vi "QR_code_Check.vi"(5 "Columns":string[](array[string]), 7 "error in (no error)":errorcluster, 8 "replace %s":string, 9 "table":string, 10 "Refnum in":T1) -> (0 "error out":errorcluster, 1 "data":string[][](array[string]), 2 "FALSE healty":bool, 3 "Refnum out":T1, 4 "TRUE Duplication on Station 2":bool)   [LabVIEW 2017]
uses:
  <vilib>/addons/database/Connection.llb/Conn ObjectReference.ctl
  <vilib>/addons/database/NI_Database_API.lvlib
panel:
  out "resulting string":string
  out "PART 1":string
  out "length 2":i32
  out "PART 2":string
  out "length":i32
  out "TRUE no barcode Done on station 1":bool
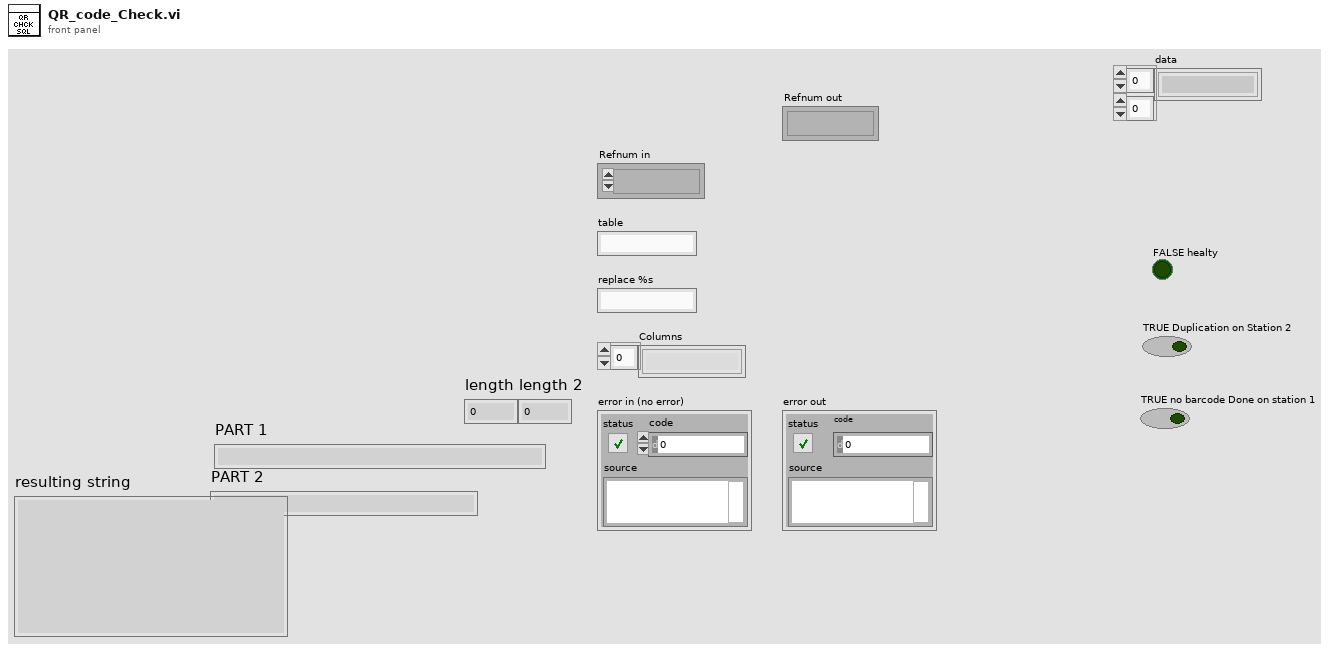
[diagram p1: front panel]
types:
  T1 = typedef "NI_Database_API.lvlib/Conn ObjectReference.ctl" = refnum<k1>
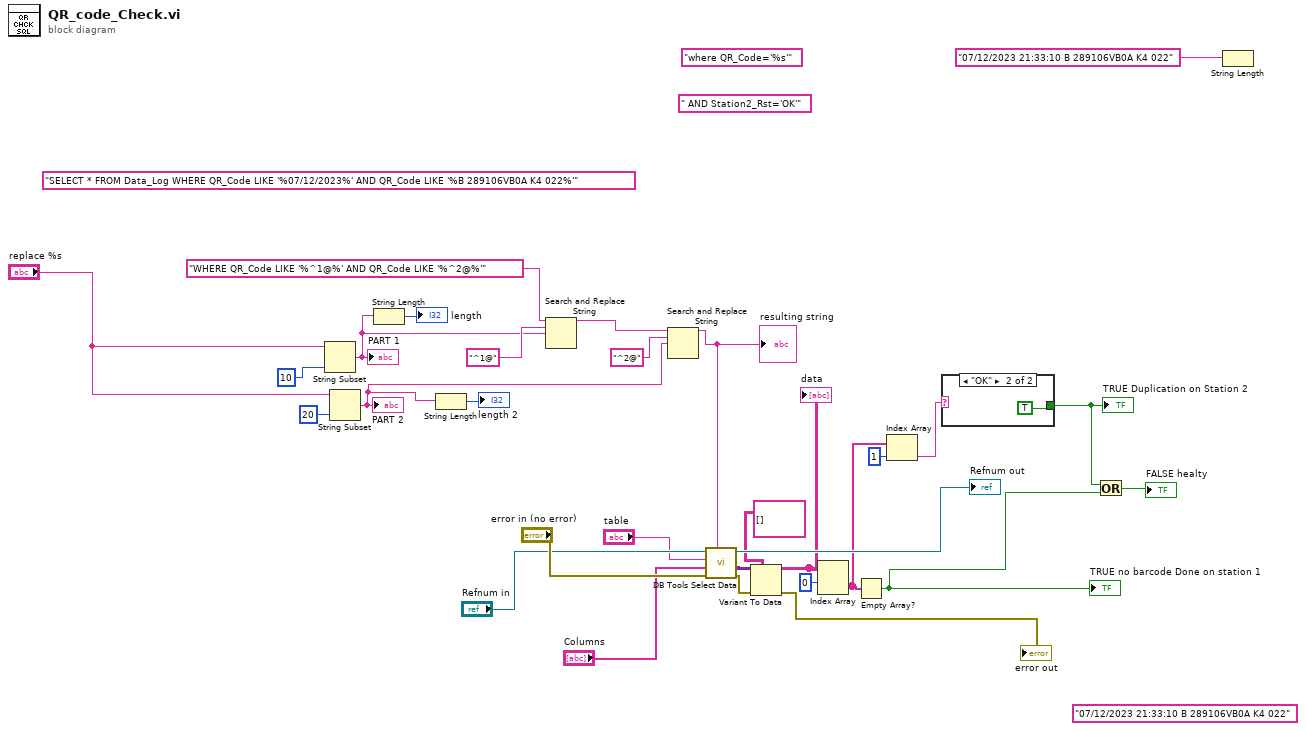
[diagram p0: block diagram]
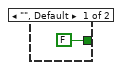
[diagram p2: hidden frame]
diagram:
  (unwired) "07/12/2023 21:33:10 B 289106VB0A K4 022" ("format string")
  (unwired) "SELECT * FROM Data_Log WHERE QR_Code LIKE '%07/12/2023%' AND QR_Code LIKE '%B 289106VB0A K4 022%'" ("format string")
  (unwired) "where QR_Code='%s'" ("format string")
  (unwired) " AND Station2_Rst='OK'" ("replace %s")
  n1 = String Subset(string="replace %s", length (rest)=10 ("offset (0)")) -> (substring=w4:string)  [unwired: 1 in]
  "PART 1" <- w4
  n2 = String Subset(string="replace %s", offset (0)=20) -> (substring=w3:string)  [unwired: 1 in]
  "PART 2" <- w3
  n3 = String Length(string=w4) -> (length=→"length":i32)
  n4 = String Length(string=w3) -> (length=→"length 2":i32)
  n5 = Search and Replace String(input string="WHERE QR_Code LIKE '%^1@%' AND QR_Code LIKE '%^2@%'" ("format string"), search string="^1@", replace string=w4) -> (result string=w7:string)  [unwired: 5 in, 3 out]
  n6 = Search and Replace String(input string=w7, search string="^2@", replace string=w3) -> (result string=w2:string)  [unwired: 5 in, 3 out]
  "resulting string" <- w2
  n7 = call <vilib>:"DB Tools Select Data.vi"("condition"=w2, "error in (no error)"="error in (no error)", "columns"="Columns", "table"="table", "connection reference"="Refnum in") -> ("error out"=w20:errorcluster, "data"=w22:variant[][], "connection reference out"=→"Refnum out":T1)  [unwired: 1 in]
  n8 = Variant To Data(error in=w20, type=string[][] [], Variant=w22) -> (data=w21:string[][], error out=→"error out":errorcluster)
  "data" <- w21
  n9 = Index Array(array=w21, index (row)=0) -> (element=w18:string[])  [unwired: 1 in]
  n10 = Empty Array?(array=w18) -> (empty?=w15:bool)
  "TRUE no barcode Done on station 1" <- w15
  n11 = Index Array(array=w18, index=1 ("index (row)")) -> (element=w17:string)
  n12 = case shown="\"OK\"" w17 {
    tunnel: [FALSE TRUE] -> w14
    frame "", Default {
    }
    frame "OK" {
    }
  }
  "TRUE Duplication on Station 2" <- w14
  n13 = Or(x=w14, y=w15) -> (x .or. y?=→"FALSE healty":bool)
  n14 = String Length(string="07/12/2023 21:33:10 B 289106VB0A K4 022" ("format string")) -> ()  [unwired: 1 out]
